vi "Alarma_EN50160_G06.vi"() -> ()   [LabVIEW 2018]
uses:
  Global/PQ_flags.vi
  Global/Alarmas_indicadores-LED.vi
  Global/estadoGeneradores.vi
  Global/Demo.vi
panel:
  in  "type specifier VI Refnum (for type only) 5":refnum<vi>
  in  "type specifier VI Refnum (for type only) 4":refnum<vi>
  in  "type specifier VI Refnum (for type only) 3":refnum<vi>
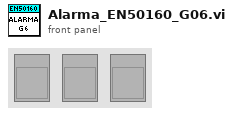
[diagram p1: front panel]
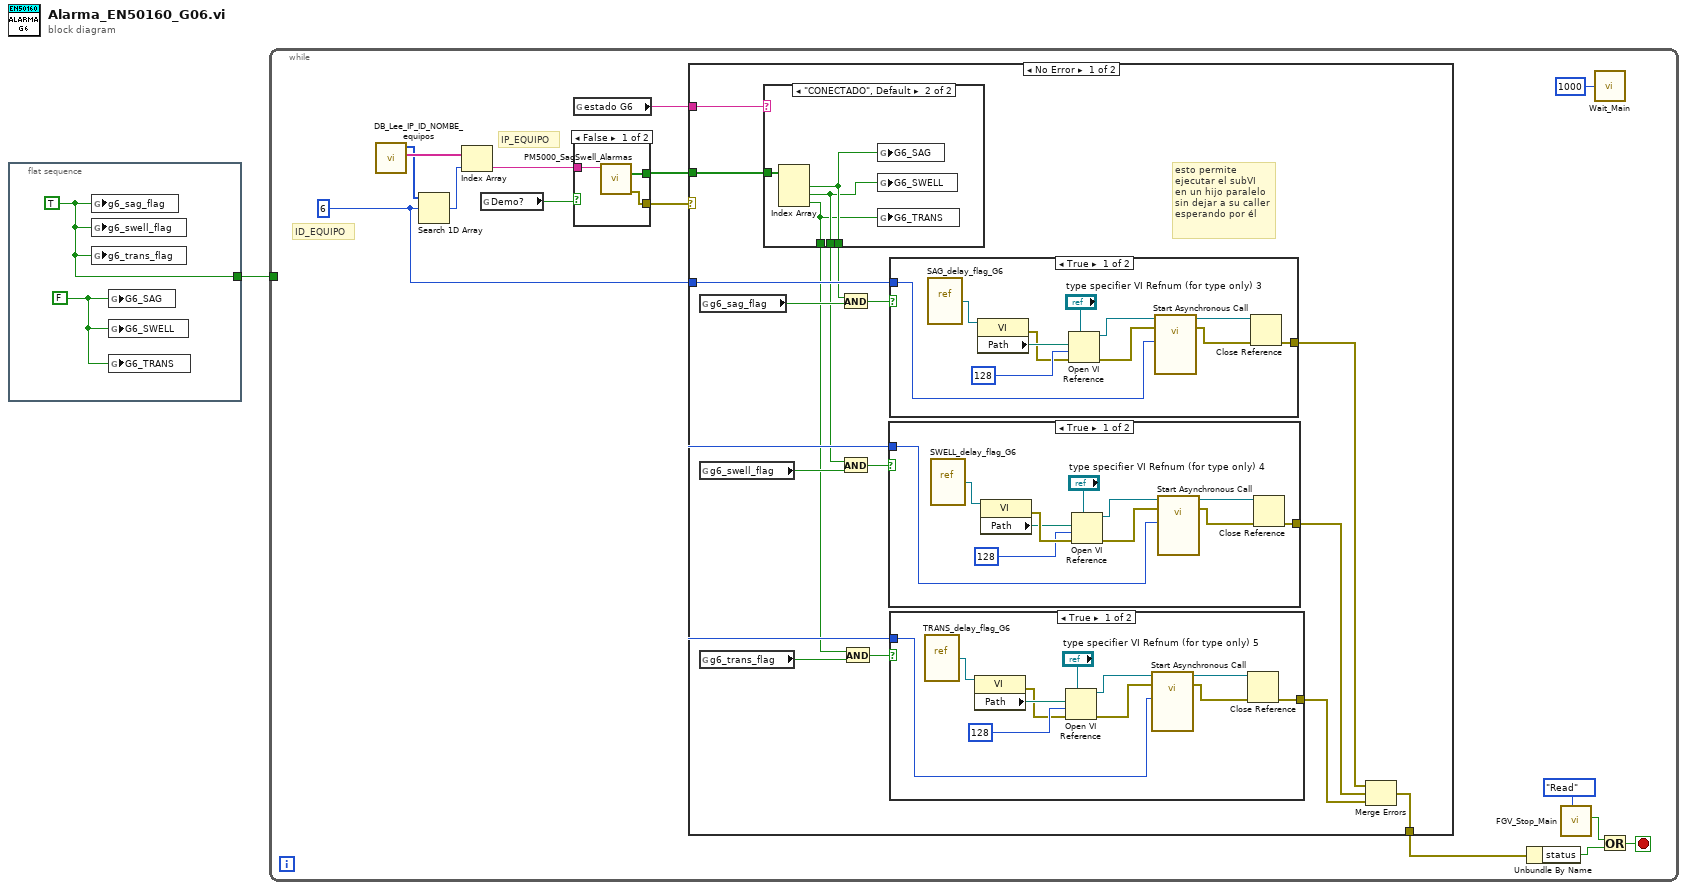
[diagram p0: block diagram]
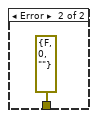
[diagram p6: hidden frame]
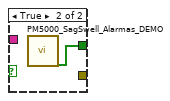
[diagram p7: hidden frame]
diagram:
  n1 = flat-sequence {
    tunnel: [w3] -> w1
    frame #0 {
      w2 = FALSE ("G1_SAG")
      w3 = TRUE ("sag_flag")
      n2 = global write "PQ_flags.vi" "g6_sag_flag"(w3) -> ()
      n3 = global write "PQ_flags.vi" "g6_swell_flag"(w3) -> ()
      n4 = global write "PQ_flags.vi" "g6_trans_flag"(w3) -> ()
      n5 = global write "Alarmas_indicadores-LED.vi" "G6_SAG"(w2) -> ()
      n6 = global write "Alarmas_indicadores-LED.vi" "G6_SWELL"(w2) -> ()
      n7 = global write "Alarmas_indicadores-LED.vi" "G6_TRANS"(w2) -> ()
    }
  }
  n8 = while {
    tunnel: w1 -> [_]
    stop <- w9 stop-if-true
    w13 = 6 ("element")
    # "IP_EQUIPO"
    # "ID_EQUIPO"
    n9 = call "DB_Lee_IP_ID_NOMBE_equipos.vi"() -> ("IP_EQUIPO"=w17:string[], "ID_EQUIPO"=w15:i32[])  [unwired: 8 in, 2 out]
    n10 = Search 1D Array(1D array=w15, element=w13) -> (index of element=w16:i32)  [unwired: 1 in]
    n11 = Index Array(array=w17, index=w16) -> (element=w14:string)
    n12 = global read "Demo.vi" "Demo?"() -> (w4:bool)
    n13 = global read "estadoGeneradores.vi" "estado G6"() -> (w10:string)
    n14 = case shown="False" w4 {
      tunnel: [w75 w76] -> w18
      tunnel: w14 -> [w74 _]
      tunnel: [w73 _] -> w5
      frame False {
        n15 = call "PM5000_SagSwell_Alarmas.vi"("Network Path"=w74) -> ("error out"=w73:errorcluster, "PQ_Alarmas"=w75:bool[])  [unwired: 8 in, 1 out]
      }
      frame True {
        n16 = call "PM5000_SagSwell_Alarmas_DEMO.vi"() -> ("PQ_Alarmas 6"=w76:bool[])  [unwired: 14 in, 5 out]
      }
    }
    n17 = case shown="No Error" w5 {
      tunnel: w18 -> [w34 _]
      tunnel: w13 -> [w27 _]
      tunnel: w10 -> [w23 _]
      tunnel: [w19 errorcluster {"status"=FALSE, "code"=0, "source"=""} ("error IO")] -> w6
      frame No Error {
        # "esto permite \nejecutar el subVI\nen un hijo paralelo\nsin dejar a su caller\nesperando por él"
        n18 = global read "PQ_flags.vi" "g6_sag_flag"() -> (w30:bool)
        n19 = global read "PQ_flags.vi" "g6_swell_flag"() -> (w29:bool)
        n20 = global read "PQ_flags.vi" "g6_trans_flag"() -> (w28:bool)
        n21 = case shown="\"CONECTADO\", Default" w23 {
          tunnel: w34 -> [_ w38]
          tunnel: [_ w37] -> w26
          tunnel: [_ w36] -> w25
          tunnel: [_ w35] -> w24
          frame "DESCONECTADO" {
          }
          frame "CONECTADO", Default {
            n22 = Index Array(array=w38) -> (element #1=w37:bool, element #2=w36:bool, element #3=w35:bool)  [unwired: 3 in]
            n23 = global write "Alarmas_indicadores-LED.vi" "G6_SAG"(w37) -> ()
            n24 = global write "Alarmas_indicadores-LED.vi" "G6_SWELL"(w36) -> ()
            n25 = global write "Alarmas_indicadores-LED.vi" "G6_TRANS"(w35) -> ()
          }
        }
        n26 = And(x=w26, y=w30) -> (x .and. y?=w33:bool)
        n27 = And(x=w25, y=w29) -> (x .and. y?=w32:bool)
        n28 = And(x=w24, y=w28) -> (x .and. y?=w31:bool)
        n29 = case shown="True" w32 {
          tunnel: w27 -> [w51 _]
          tunnel: [w50 _] -> w21
          frame True {
            n30 = vi-ref "SWELL_delay_flag_G6.vi"() -> (w58:refnum<vi>)
            n31 = property class="VI"(reference=w58) -> (error out=w60:errorcluster, "Path"=w59:path)  [unwired: 1 in, 1 out]
            n32 = Open VI Reference(type specifier VI Refnum (for type only)="type specifier VI Refnum (for type only) 4", vi path=w59, options=128, error in (no error)=w60) -> (vi reference=w56:refnum<vi>, error out=w52:errorcluster)  [unwired: 2 in]
            n33 = call-by-ref "Start Asynchronous Call"(reference=w56, error in=w52, "ID_EQUIPO"=w51) -> (reference out=w53:refnum<vi>, error out=w54:errorcluster)  [unwired: 11 in]
            n34 = Close Reference(reference=w53, error in (no error)=w54) -> (error out=w50:errorcluster)
          }
          frame False {
          }
        }
        n35 = case shown="True" w33 {
          tunnel: w27 -> [w62 _]
          tunnel: [w61 _] -> w22
          frame True {
            n36 = vi-ref "SAG_delay_flag_G6.vi"() -> (w65:refnum<vi>)
            n37 = property class="VI"(reference=w65) -> (error out=w63:errorcluster, "Path"=w64:path)  [unwired: 1 in, 1 out]
            n38 = Open VI Reference(type specifier VI Refnum (for type only)="type specifier VI Refnum (for type only) 3", vi path=w64, options=128, error in (no error)=w63) -> (vi reference=w67:refnum<vi>, error out=w71:errorcluster)  [unwired: 2 in]
            n39 = call-by-ref "Start Asynchronous Call"(reference=w67, error in=w71, "ID_EQUIPO"=w62) -> (reference out=w70:refnum<vi>, error out=w69:errorcluster)  [unwired: 11 in]
            n40 = Close Reference(reference=w70, error in (no error)=w69) -> (error out=w61:errorcluster)
          }
          frame False {
          }
        }
        n41 = case shown="True" w31 {
          tunnel: w27 -> [w40 _]
          tunnel: [w39 _] -> w20
          frame True {
            n42 = vi-ref "TRANS_delay_flag_G6.vi"() -> (w43:refnum<vi>)
            n43 = property class="VI"(reference=w43) -> (error out=w41:errorcluster, "Path"=w42:path)  [unwired: 1 in, 1 out]
            n44 = Open VI Reference(type specifier VI Refnum (for type only)="type specifier VI Refnum (for type only) 5", vi path=w42, options=128, error in (no error)=w41) -> (vi reference=w45:refnum<vi>, error out=w49:errorcluster)  [unwired: 2 in]
            n45 = call-by-ref "Start Asynchronous Call"(reference=w45, error in=w49, "ID_EQUIPO"=w40) -> (reference out=w48:refnum<vi>, error out=w47:errorcluster)  [unwired: 11 in]
            n46 = Close Reference(reference=w48, error in (no error)=w47) -> (error out=w39:errorcluster)
          }
          frame False {
          }
        }
        n47 = Merge Errors(w22, w21, w20) -> (w19:errorcluster)
      }
      frame Error {
      }
    }
    n48 = Unbundle By Name(w6) -> ("status"=w7:bool)
    n49 = call "FGV_Stop_Main.vi"("Action"=enum16{"Read", "Write"}."Read") -> ("Var Out"=w8:bool)  [unwired: 9 in, 1 out]
    n50 = call "Wait_Main.vi"("Wait time (msec)"=u32 1000) -> ()  [unwired: 5 in]
    n51 = Or(x=w8, y=w7) -> (x .or. y?=w9:bool)
  }
